vi "IMAQ FPGA Camera Link 4 Tap 10-Bit.vi"(6 "Ready for Output":bool=TRUE, 7 "Camera Link Enables":T3, 8 "Cancel Acquisition":bool, 9 "Acquire":bool=TRUE, 10 "Camera Link Data":T2, 11 "Acquisition Settings":T4) -> (0 "Output Valid":bool, 2 "Acquisition Status":T1, 3 "Vision Pixel Bus Out":T5={"Pixel Data"=[0, 0, 0, 0, 0, 0, 0, 0], "DV"=[FALSE, FALSE, FALSE, FALSE, FALSE, FALSE, FALSE, FALSE], "EOL"=FALSE, "EOI"=FALSE, "Data Type"=enum."U16 x 8"}, 5 "Acquisition Overflow":bool)   [LabVIEW 2017]
doc: "Acquires images from an 4 tap 10-bit (1X4-1Y) Camera Link Camera. On each pixel clock, 4 adjacent pixels arrive starting at the left of the image. Ensure that this VI is called from a Single Cycle Timed Loop that is running faster than the pixel clock of the camera.\n\nThe <B>Vision Pixel Bus Out</B> can be connected to Vision FPGA algorithms for processing."
uses:
  <vilib>/visionFPGA/Controls/IMAQ FPGA Pixel Bus u16x8.ctl
  <vilib>/visionFPGA/Basics/Camera Link Acquisition/CL Data to Pixels/IMAQ FPGA Camera Link Data to Pixels 4 Tap 10-Bit.vi
  <vilib>/visionFPGA/Basics/Camera Link Acquisition/Pixel Packer/IMAQ FPGA Camera Link Pixel Packer U16x4.vi
  <vilib>/visionFPGA/Basics/Camera Link Acquisition/Pixel Bus to Vision Pixel Bus/IMAQ FPGA Camera Link Pixel Bus to Vision Pixel Bus U16x8.vi
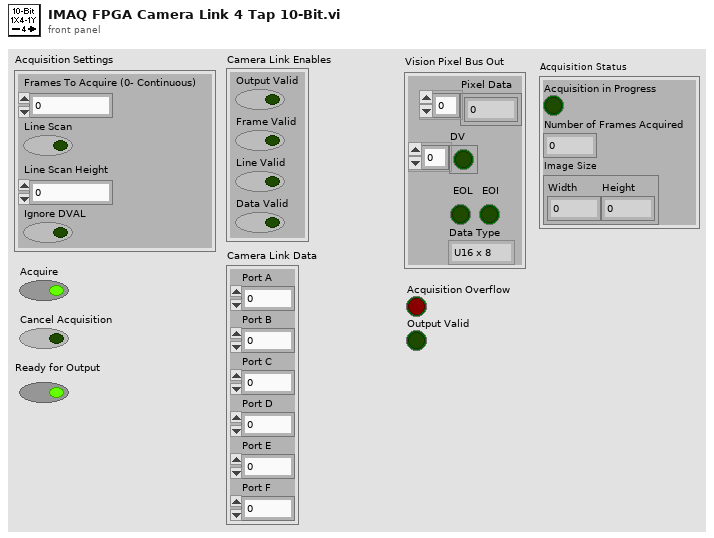
[diagram p1: front panel]
types:
  T1 = cluster{"Acquisition in Progress":bool, "Number of Frames Acquired":u32, "Image Size":cluster{"Width":u32, "Height":u32}}
  T2 = cluster{"Port A":u8, "Port B":u8, "Port C":u8, "Port D":u8, "Port E":u8, "Port F":u8}
  T3 = cluster{"Output Valid":bool, "Frame Valid":bool, "Line Valid":bool, "Data Valid":bool}
  T4 = cluster{"Frames To Acquire (0- Continuous)":u32, "Line Scan":bool, "Line Scan Height":u32, "Ignore DVAL":bool}
  T5 = typedef "IMAQ FPGA Pixel Bus u16x8.ctl" = cluster{"Pixel Data":u16[], "DV":bool[], "EOL":bool, "EOI":bool, "Data Type":enum16{"U16 x 8"}}
  T6 = cluster{"Acquisition in Progress":bool, "Num Frames Acquired":u32, "Height":u32, "Number of Cycles per Line":u32}
  T7 = cluster{"Acquisition in Progress":bool, "Num Frames Acquired":u32, cluster{u32, "Height":u32}}
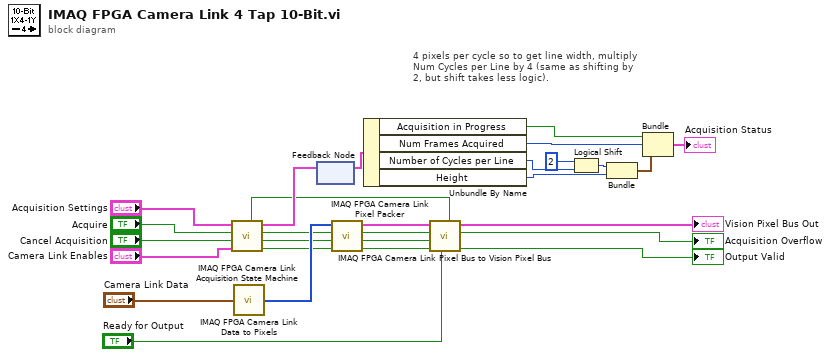
[diagram p0: block diagram]
diagram:
  # "4 pixels per cycle so to get line width, multiply Num Cycles per Line by 4 (same as shifting by 2, but shift takes less logic)."
  n1 = call <vilib>:"IMAQ FPGA Camera Link Acquisition State Machine.vi"("Enables"="Camera Link Enables", "Cancel Acq"="Cancel Acquisition", "Acquire"="Acquire", "Acquisition Settings"="Acquisition Settings") -> ("Output Valid"=w7:bool, "Frame Valid"=w8:bool, "Line Valid"=w9:bool, "Acquisition Status"=w18:T6, "Reset"=w6:bool)  [unwired: 3 in]
  n2 = call-poly <vilib>:"IMAQ FPGA Camera Link Data to Pixels.vi"("Camera Link Data"="Camera Link Data") -> ("Pixels"=w10:u16[])
  n3 = feedback #1() -> (w5:T6)  [unwired: 1 in]
  n4 = feedback-in #1(w18) -> ()
  n5 = call-poly <vilib>:"IMAQ FPGA Camera Link Pixel Packer.vi"("Input Valid"=w7, "Frame Valid In"=w8, "Line Valid In"=w9, "Pixels In"=w10) -> ("Output Valid"=w11:bool, "Frame Valid Out"=w13:bool, "Line Valid Out"=w12:bool, "Pixel Bus x8 Out"=w14:cluster{"Pixels":u16[], "DV":bool[]})  [unwired: 4 in]
  n6 = Unbundle By Name(w5) -> ("Acquisition in Progress"=w4:bool, "Num Frames Acquired"=w3:u32, "Number of Cycles per Line"=w24:u32, "Height"=w28:u32)
  n7 = call-poly <vilib>:"IMAQ FPGA Camera Link Pixel Bus to Vision Pixel Bus.vi"("Reset Overflow"=w6, "Ready for Output"="Ready for Output", "Input Valid"=w11, "Frame Valid In"=w13, "Line Valid In"=w12, "Pixel Bus x8 In"=w14) -> ("Output Valid"=→"Output Valid":bool, "Acquisition Overflow"=→"Acquisition Overflow":bool, "Vision Pixel Bus Out"=→"Vision Pixel Bus Out":T5)  [unwired: 3 in]
  n8 = Logical Shift(y=i16 2, x=w24) -> (x << y=w23:u32)
  n9 = Bundle(w23, "Height"=w28) -> (w2:cluster{u32, "Height":u32})  [unwired: 1 in]
  n10 = Bundle("Acquisition in Progress"=w4, "Num Frames Acquired"=w3, w2) -> (→"Acquisition Status":T7)  [unwired: 1 in]
